vi "Wysylanie UDP do SbRIO.vi"(7 "Cluster":T1, 8 "error in queue":errorcluster, 11 "queue in":refnum<queue>) -> (0 "error out queue":errorcluster, 1 "error out udp":errorcluster, 2 "queue out 2":refnum<queue>, 3 "connection ID out":refnum<k16>, 4 "stop error ?":bool)   [LabVIEW 2014]
uses:
  Program Files (x86)/National Instruments/LabVIEW 2014/examples/Design Patterns/Queued Message Handler/support/QMH Fundamentals - Message Cluster.ctl
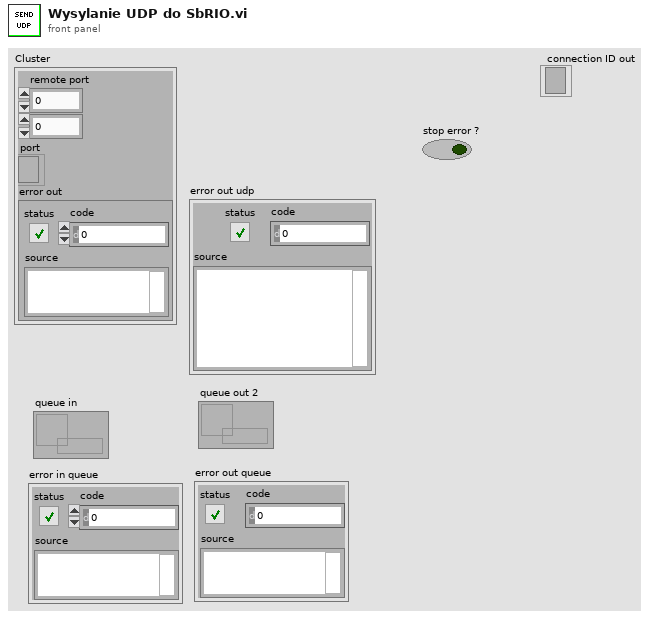
[diagram p1: front panel]
types:
  T1 = cluster{"remote port":u16, u32, "port":refnum<k16>, "error out":errorcluster}
  T2 = typedef "QMH Fundamentals - Message Cluster.ctl" = cluster{"Message":string, "Message Data":variant}
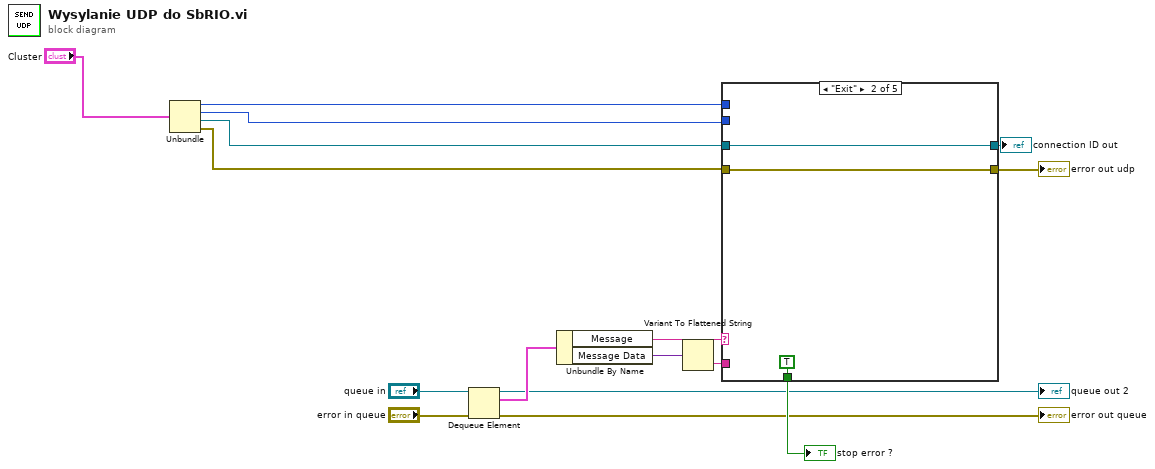
[diagram p0: block diagram]
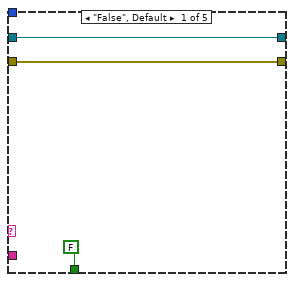
[diagram p2: hidden frame]
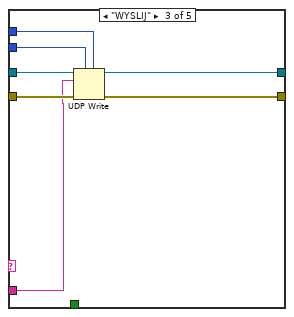
[diagram p3: hidden frame]
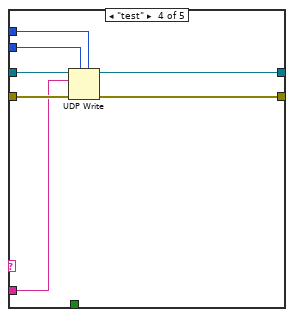
[diagram p4: hidden frame]
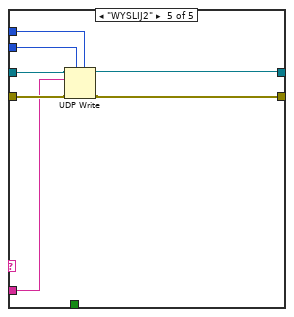
[diagram p5: hidden frame]
diagram:
  n1 = Unbundle("Cluster") -> ("remote port"=w7:u16, w8:u32, "port"=w6:refnum<k16>, "error out"=w5:errorcluster)
  n2 = Dequeue Element(queue="queue in", error in (no error)="error in queue") -> (queue out=→"queue out 2":refnum<queue>, element=w11:T2, error out=→"error out queue":errorcluster)  [unwired: 1 in, 1 out]
  n3 = Unbundle By Name(w11) -> ("Message"=w12:string, "Message Data"=w1:variant)
  n4 = Variant To Flattened String(Variant=w1) -> (data string=w4:string)  [unwired: 1 out]
  n5 = case shown="\"Exit\"" w12 {
    tunnel: w8 -> [_ _ w25 w33 w38]
    tunnel: w7 -> [_ _ w24 w34 w37]
    tunnel: w6 -> [w17 w20 w26 w32 w41]
    tunnel: w5 -> [w19 w22 w29 w31 w42]
    tunnel: [w19 w22 w28 w36 w43] -> w9
    tunnel: [FALSE TRUE _ _ _] -> w16
    tunnel: w4 -> [_ _ w23 w30 w40]
    tunnel: [w17 w20 w27 w35 w39] -> w2
    frame "False", Default {
    }
    frame "Exit" {
    }
    frame "WYSLIJ" {
      n6 = UDP Write(address=w25, port or service name=w24, connection ID=w26, data in=w23, 8:w29) -> (error out=w28:errorcluster, 3:w27:refnum<k16>)  [unwired: 1 in]
    }
    frame "test" {
      n7 = UDP Write(address=w33, port or service name=w34, connection ID=w32, data in=w30, 8:w31) -> (error out=w36:errorcluster, 3:w35:refnum<k16>)  [unwired: 1 in]
    }
    frame "WYSLIJ2" {
      n8 = UDP Write(address=w38, port or service name=w37, connection ID=w41, data in=w40, 8:w42) -> (error out=w43:errorcluster, 3:w39:refnum<k16>)  [unwired: 1 in]
    }
  }
  "stop error ?" <- w16
  "error out udp" <- w9
  "connection ID out" <- w2
